vi "Martins HOT interface.vi"() -> ()   [LabVIEW 2011]
uses:
  Sub VIs/Trap cluster.ctl
  <vilib>/Utility/inputDevices.llb/closeKeyboard.vi
  <vilib>/Utility/inputDevices.llb/keyboardAcquire.vi
  <vilib>/Utility/file.llb/Write To Spreadsheet File (DBL).vi
  <vilib>/vision/driver/NI_Vision_Acquisition_Software.lvlib
panel:
  in  "e_desired":sgl=0.5
  in  "Apply Corrections":bool
  in  "View Licence":bool
  in  "ok":bool caption="Mark the center of \nthe spot using the \nzoom and the point\ntool, then click this \nbutton"
  in  "Stop program":bool
  in  "Updating trap cluster":bool=TRUE
  out "Camera enabled":bool
  out "SLM enabled":bool
  in  "Run calibration":bool
  in  "Hologram generation":cluster{"Method":i32, "Iterations":i32}={"Method"=0, "Iterations"=10} {"Method" items=["Lenses & Gratings (3D)", " Gerchberg-Saxton (3D)", "Gerchberg-Saxton FFT (2D)"]}
  in  "Show image":bool=TRUE
  in  "Follow traps":bool=TRUE
  in  "Purge data":bool
  in  "ROI size":dbl=2.0 min=2.0 step=2.0
  in  "Save data":bool
  in  "Video tracking":bool
  in  "Display hologram\nand computed \nimage plane":bool
  in  "ROI":T1={"Global Rectangle"=[309, 286, 371, 364], "Contours"=[{"Contour Type"=0, "ROI Type"=1, "Points"=[370, 286]}, {"Contour Type"=0, "ROI Type"=1, "Points"=[351, 363]}, {"Contour Type"=0, "ROI Type"=1, "Points"=[309, 315]}]}
  out "Image":T2(plugin-control)
  out "Calculated image plane":dbl[][](graph)
  in  "G":bool[](array[boolean])=[FALSE, FALSE, FALSE]
  out "Current trap pos":T3={"X (IMAQ)"=[57.0, 561.4247207088292, 45.0], "Y (IMAQ)"=[160.0, 450.3470670604607, 127.0], "Z"=[0.0, 0.0, 0.0], "Amplitudes"=[10.0, 10.0, 10.0], "Trap number"=[0, 1, 2], "ROI number"=[0, 1, 2], "Number of traps"=3, "Group"=[]}
  out "NI Vision error":errorcluster
  out "CUDA/SLM error":errorcluster
  in  "Cancel calibration":bool
  in  "Skip step if \ntimed out":bool
  in  "Display path":bool=TRUE
  out "Average step time (ms)":dbl
  in  "Step time \n(ms)":u32=10
  in  "Pause":bool
  in  "cancel path":bool
  out "Step skipped":bool
  in  "Path controls":T4={"follow path"=FALSE, "Step length"=1.0, "Arrive \nsimultaneously"=TRUE, "Synchronize traps"=FALSE, "Add current \npositions to path"=FALSE}
  in  "Create path":bool
  out "#":i32[](array[numeric])=[0, 1, 2]
  in  "Group \nTraps":bool
  in  "Move \nHandle":bool
  out "Displayed Hologram":u8[][](graph)
  in  "Coordinate mapping \n(IMAQ to SLM)":T5={"sX"=-256.0, "sY"=-256.0, "sZ"=0.0, "cX"=0.5, "cY"=0.5, "cZ"=1.0}
  in  "Switch X/Y":bool
  in  "I":dbl[](array[numeric])=[10.0, 10.0, 10.0]
  in  "Z":dbl[](array[numeric])=[0.0, 0.0, 0.0]
  # "Martin\nPersson 2011"
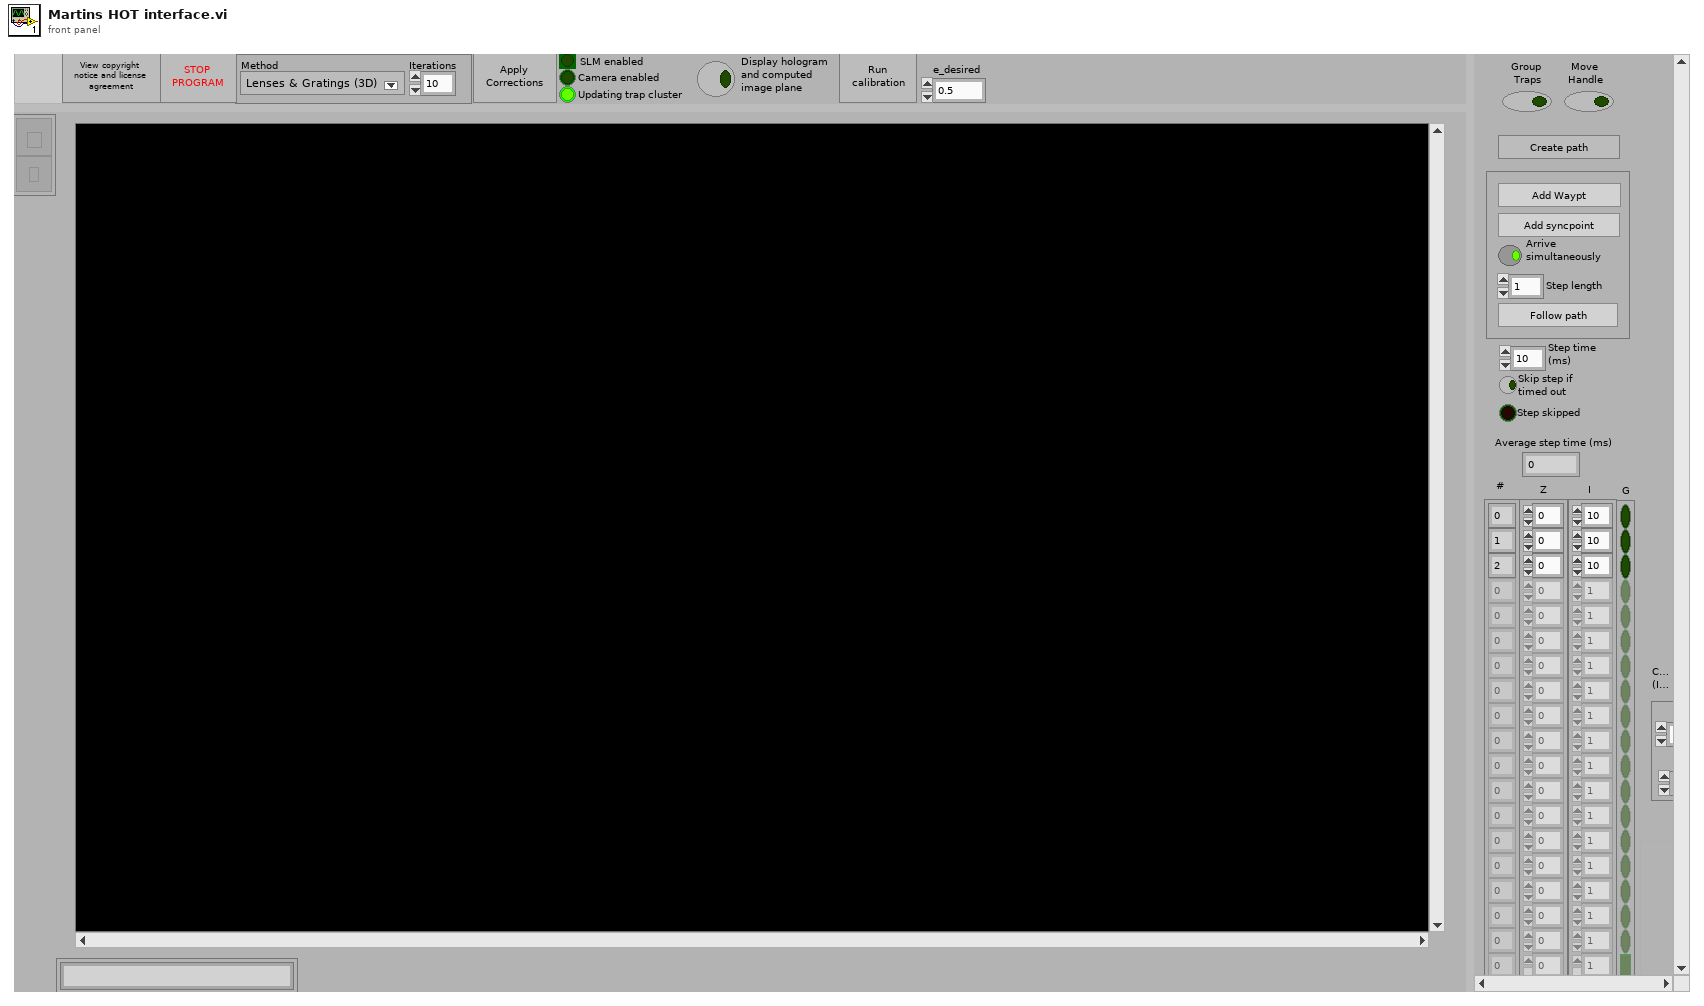
[diagram p1: front panel]
types:
  T1 = cluster{"Global Rectangle":i32[], "Contours":cluster{"Contour Type":u32, "ROI Type":u32, "Points":i32[]}[]}
  T2 = typedef "IMAQ Image.ctl" = refnum<image>
  T3 = typedef "Trap cluster.ctl" = cluster{"X (IMAQ)":dbl[], "Y (IMAQ)":dbl[], "Z":dbl[], "Amplitudes":dbl[], "Trap number":i32[], "ROI number":i32[], "Number of traps":i32, "Group":bool[]}
  T4 = cluster{"follow path":bool, "Step length":dbl, "Arrive \nsimultaneously":bool, "Synchronize traps":bool, "Add current \npositions to path":bool}
  T5 = cluster{"sX":dbl, "sY":dbl, "sZ":dbl, "cX":dbl, "cY":dbl, "cZ":dbl}
  T6 = cluster{"Centroid X":dbl[], "Centroid Y":dbl[], "Acquired Buffer Number":u32}
  T7 = typedef "IMAQdx.ctl" = refnum<k21>
  T8 = typedef "Image Type" = u32
  T9 = enum16{"0", "1", "2", "3", "4", "5", "6", "7", "8", "9", "A", "B", "C", "D", "E", "F", "G", "H", "I", "J", "K", "L", "M", "N", "O", "P", "Q", "R", "S", "T", "U", "V", "W", "X", "Y", "Z", "F1", "F2", "F3", "F4", "F5", "F6", "F7", "F8", "F9", "F10", "F11", "F12", "F13", "F14", "F15", "ADD", "BACK", "BACKSLASH", "CAPITAL", "COMMA", "DECIMAL", "DELETE", "DIVIDE", "DOWN", "END", "EQUALS", "ESCAPE", "GRAVE (`)", "HOME", "INSERT", "LBRACKET", "LCONTROL", "LEFT", "L ALT", "LSHIFT", "LWIN", "MINUS", "MULTIPLY", "NEXT", "NUMLOCK", "NUMPAD_0", "NUMPAD_1", "NUMPAD_2", "NUMPAD_3", "NUMPAD_4", "NUMPAD_5", "NUMPAD_6", "NUMPAD_7", "NUMPAD_8", "NUMPAD_9", "PAUSE", "PERIOD", "PRIOR (PG UP)", "RBRACKET", "RCONTROL", "RETURN", "RIGHT", "R ALT", "RSHIFT", "RWIN", "SCROLL", "SEMICOLON", "SLASH", "SPACE", "SUBTRACT", "TAB", "UP", "ENTER (num pad)", "' (quote)"}[]
  T10 = typedef "LVRectTypeDef.ctl" = cluster{"left":i16, "top":i16, "right":i16, "bottom":i16}
  T11 = cluster{dbl[], dbl[], "Acquired Buffer Number":u32}
  T12 = cluster{"Centroid X":dbl[], "Centroid Y":dbl[], "Acquired Buffer Number":u32}[]
  T13 = cluster{"Contour Type":u32, "ROI Type":u32, "Points":i32[]}[]
  T14 = cluster{"Contour Type":u32, "ROI Type":u32, "Points":i32[]}
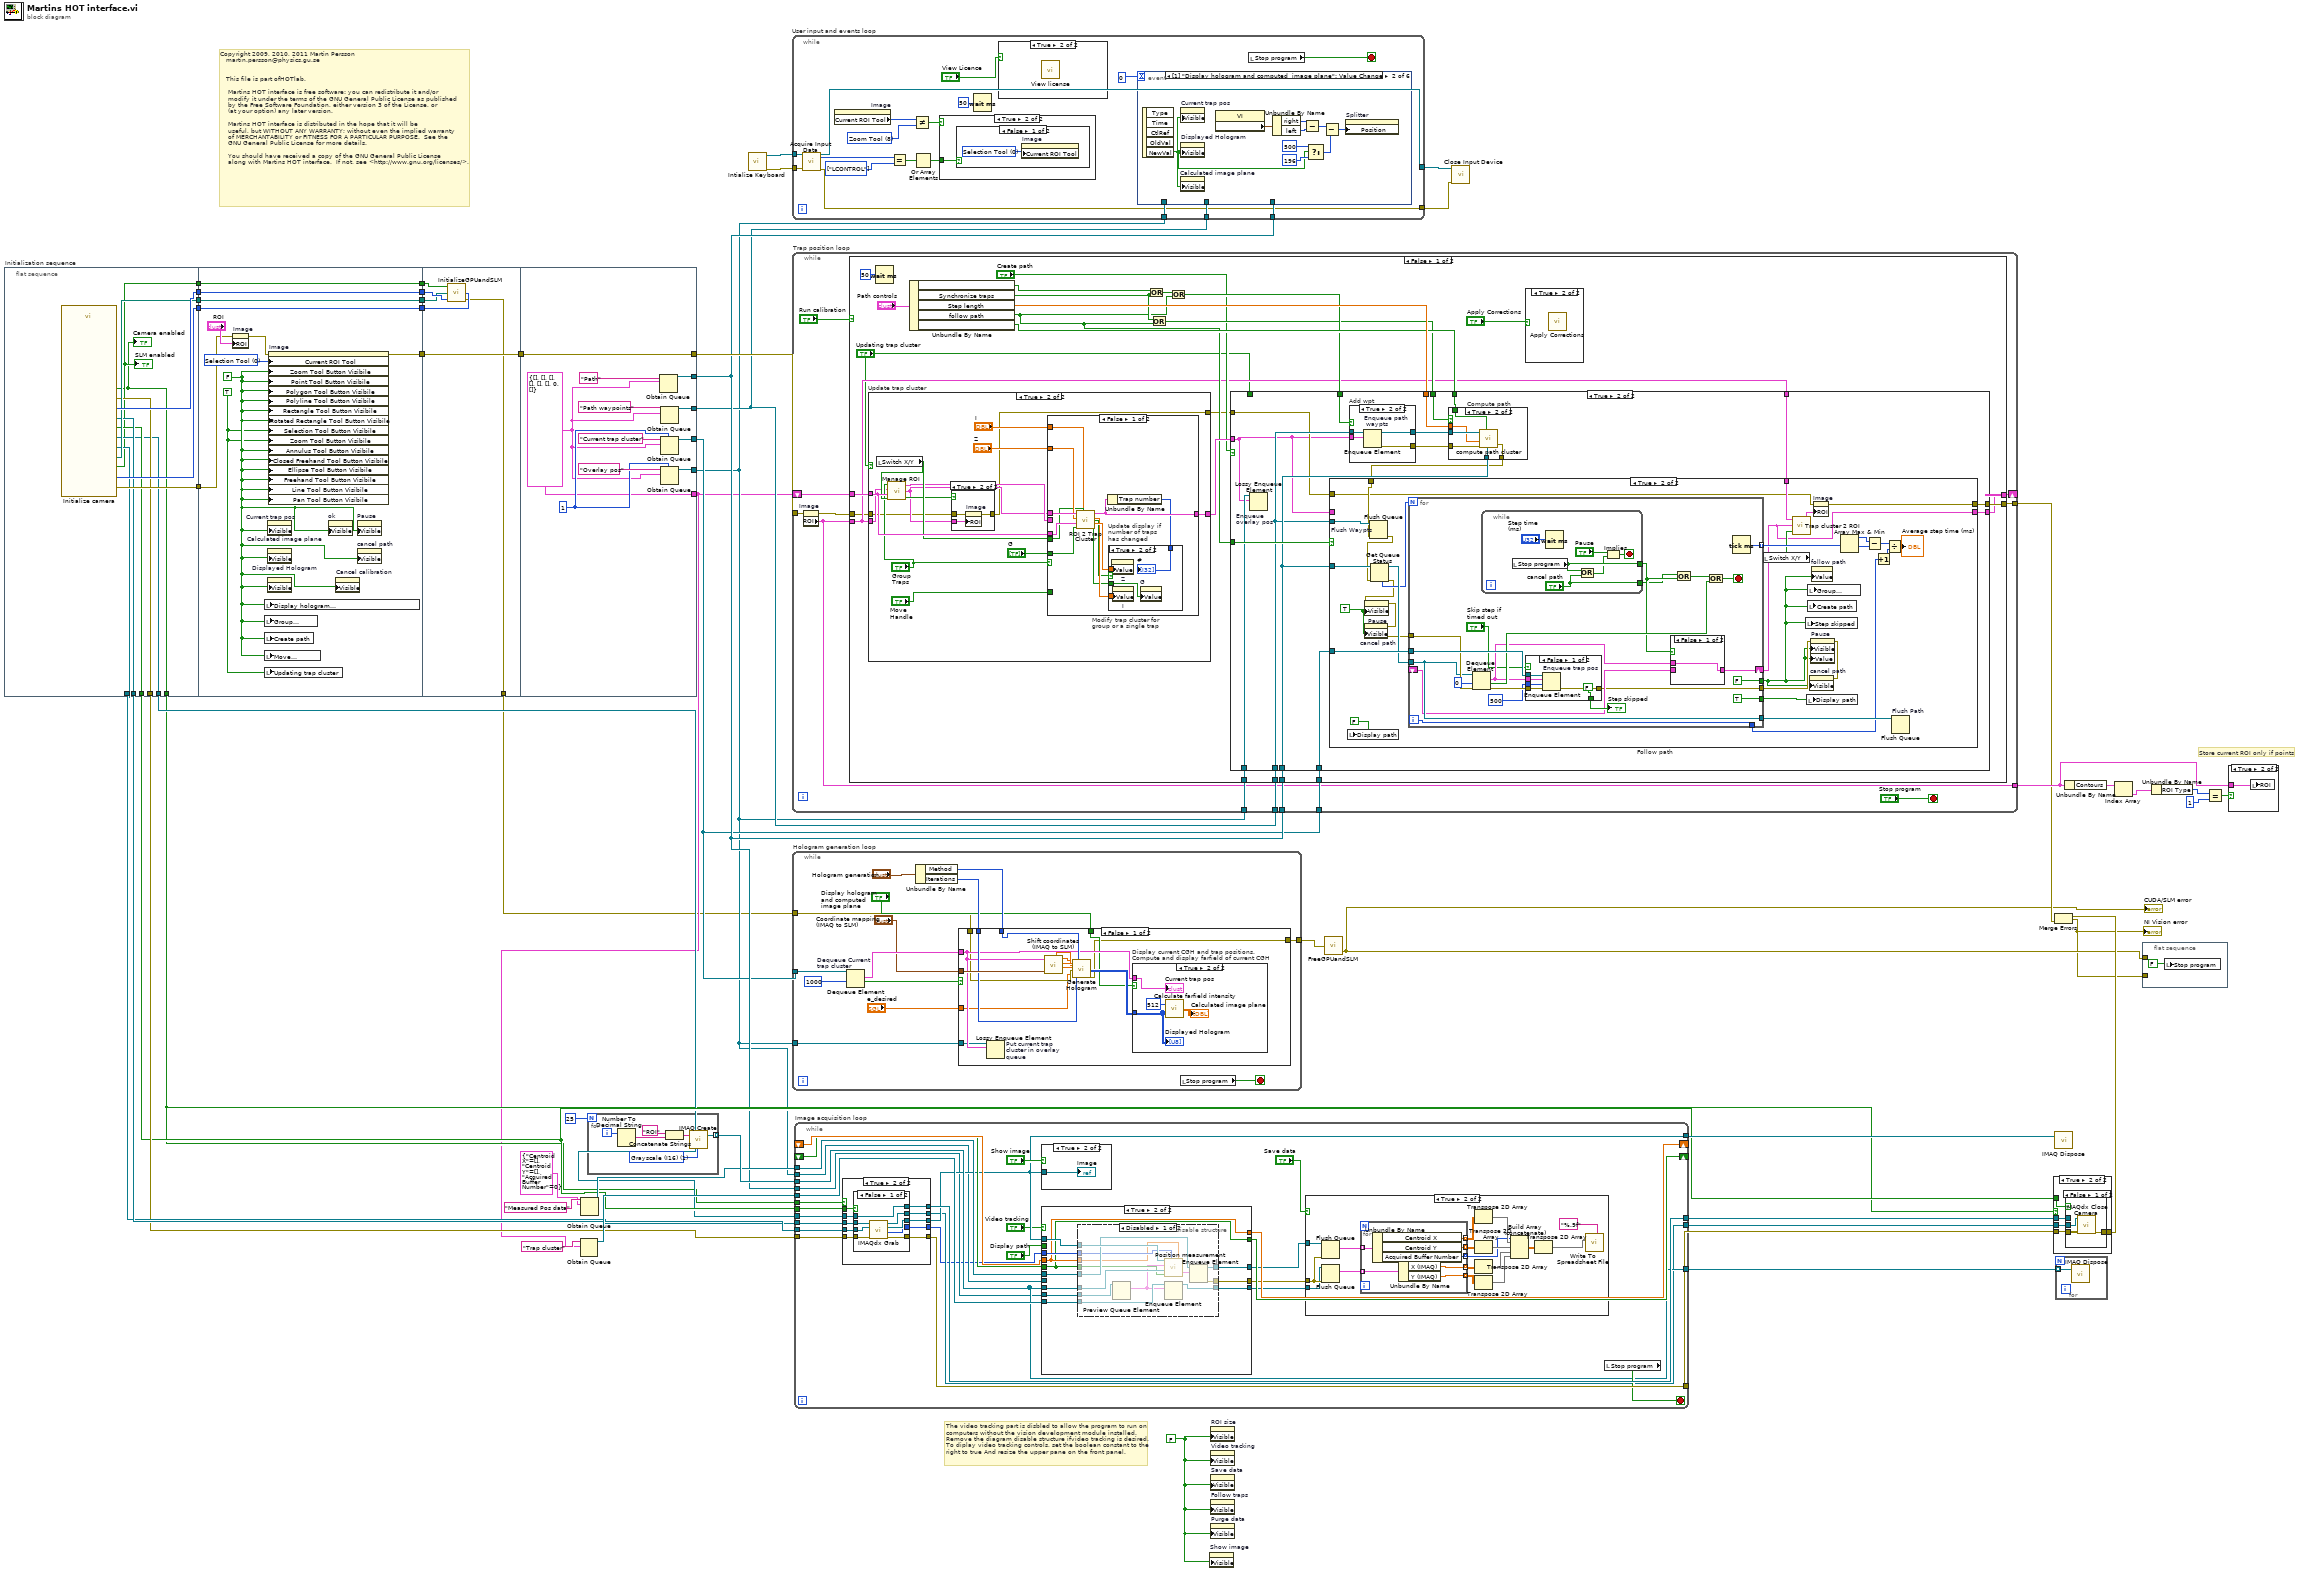
[diagram p0: block diagram]
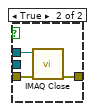
[diagram p3: hidden frame]
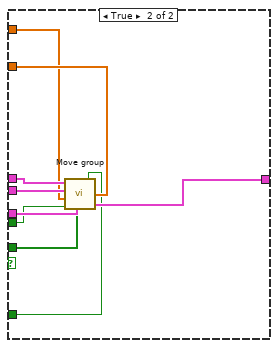
[diagram p10: hidden frame]
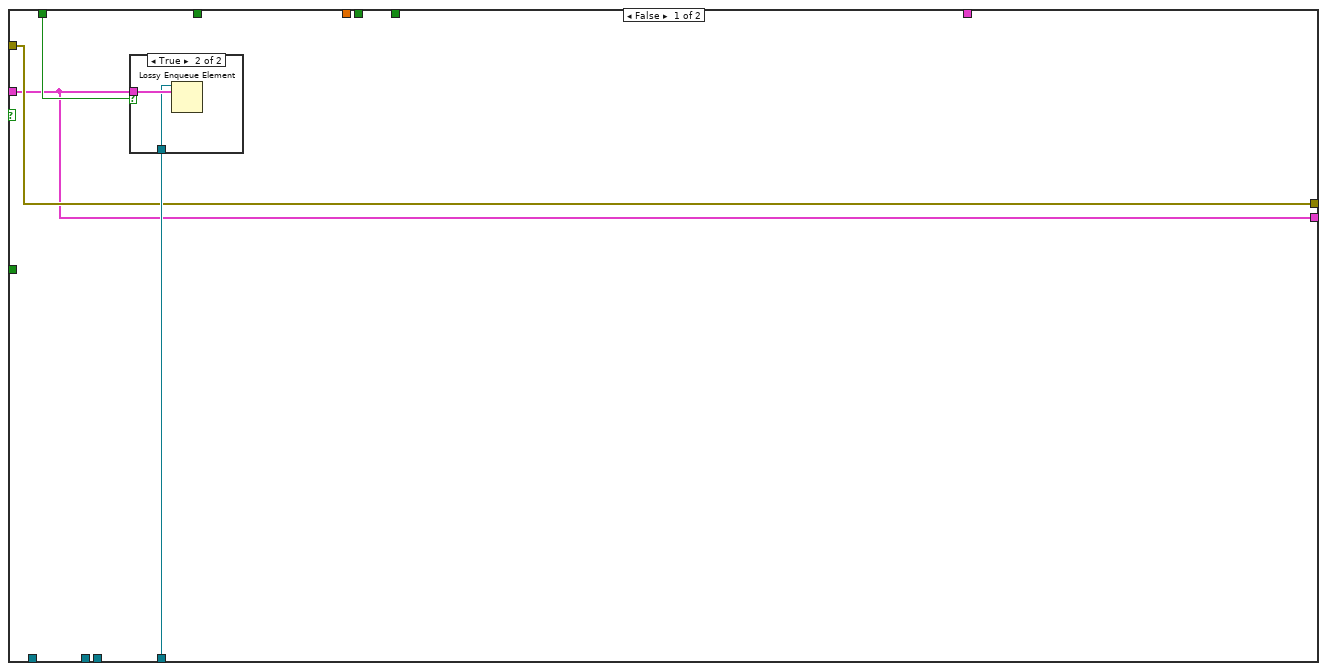
[diagram p11: hidden frame]
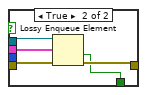
[diagram p14: hidden frame]
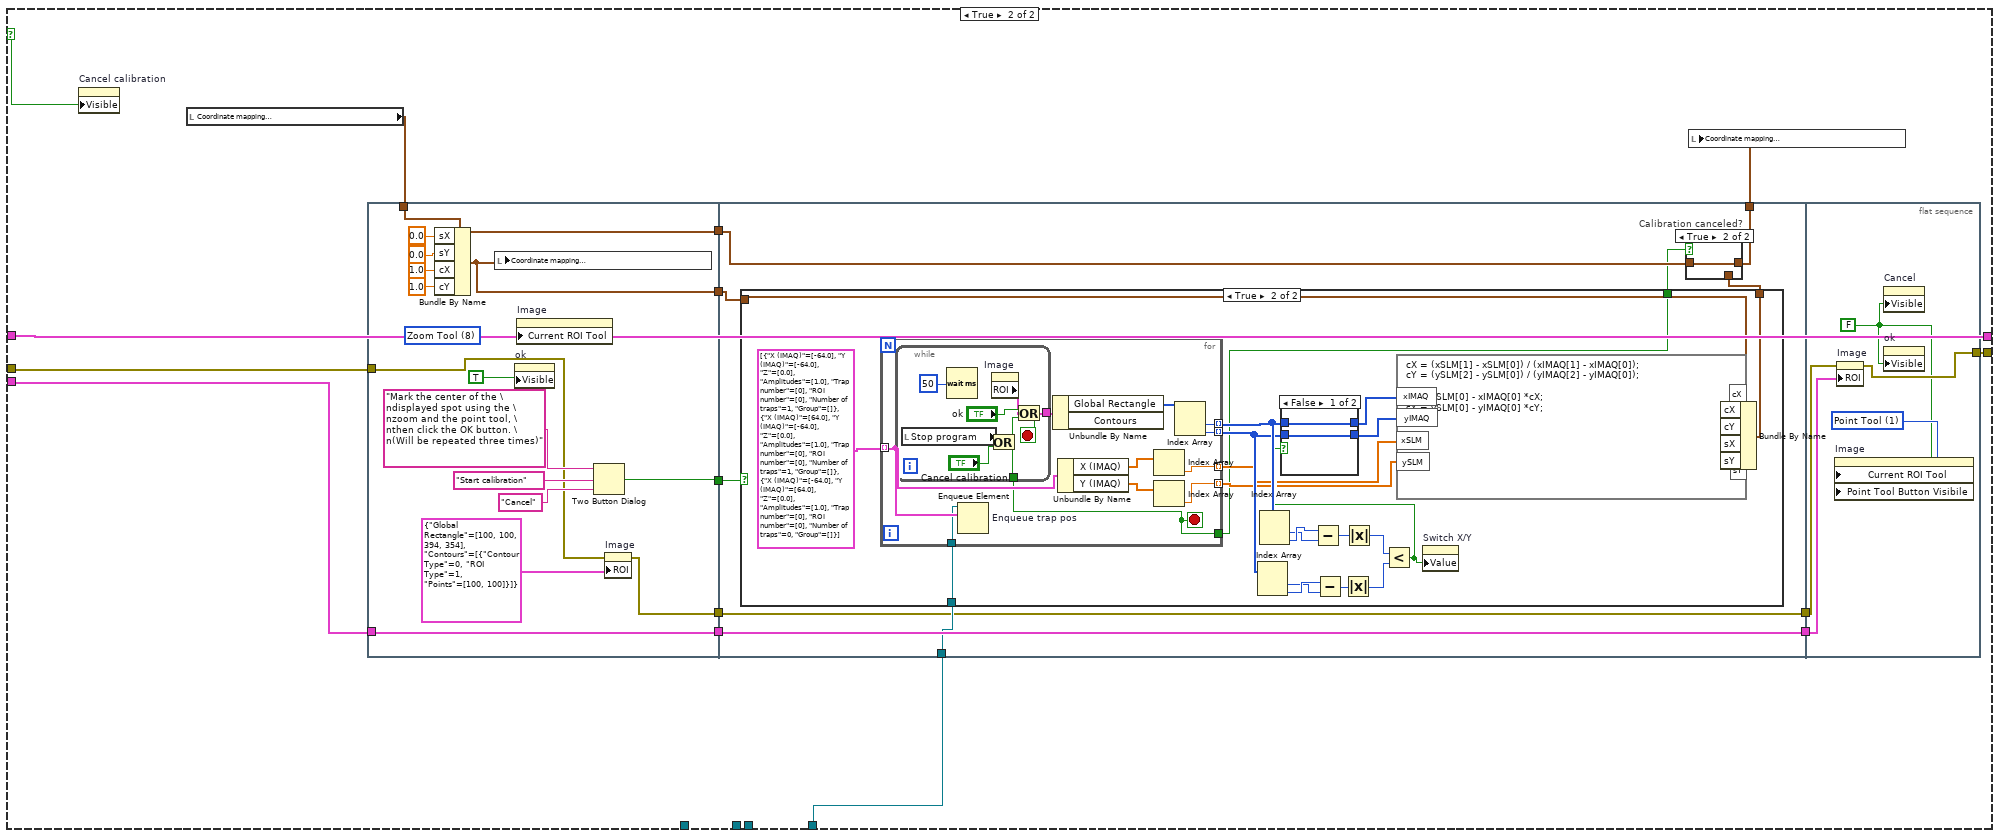
[diagram p18: hidden frame]
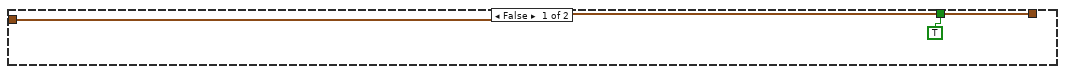
[diagram p20: hidden frame]
diagram:
  w39 = FALSE ("Visible")
  # "Copyright 2009, 2010, 2011 Martin Persson \n   martin.persson@physics.gu.se\n\n\n   This file is part ofHOTlab.\n\n    Martins HOT interface is free software: you can redistribute it and/or \n    modify it under the terms of the GNU General Public License as published \n    by the Free Software Foundation, either version 3 of the License, or\n    (at your option) any later version.\n\n    Martins HOT interface is distributed in the hope that it will be \n    useful, but WITHOUT ANY WARRANTY; without even the implied warranty\n    of MERCHANTABILITY or FITNESS FOR A PARTICULAR PURPOSE.  See the\n    GNU General Public License for more details.\n\n    You should have received a copy of the GNU General Public License\n    along with Martins HOT interface.  If not, see <http://www.gnu.org/licenses/>."
  # "Store current ROI only if points"
  # "The video tracking part is disbled to allow the program to run on\ncomputers without the vision development module installed. \nRemove the diagram disable structure ifvideo tracking is desired. \nTo diplay video tracking controls, set the boolean constant to the \nright to true And resize the upper pane on the front panel."
  n1 = flat-sequence "Initialization sequence" {
    tunnel: [w54] -> w24
    tunnel: [w63] -> w23
    tunnel: [w62] -> w22
    tunnel: [w61] -> w21
    tunnel: [w60] -> w20
    tunnel: [w59] -> w18
    tunnel: [w58] -> w17
    tunnel: [w57] -> w16
    tunnel: [w56] -> w15
    tunnel: [w55] -> w14
    tunnel: [w53] -> w13
    tunnel: w24 -> [w71]
    tunnel: w23 -> [w69]
    tunnel: w22 -> [w74]
    tunnel: w21 -> [w73]
    tunnel: w20 -> [w72]
    tunnel: [w71] -> w7
    tunnel: [w64] -> w6
    tunnel: [w74] -> w4
    tunnel: [w73] -> w3
    tunnel: [w72] -> w2
    tunnel: w7 -> [w77]
    tunnel: w6 -> [w80]
    tunnel: [w80] -> w5
    tunnel: w4 -> [w78]
    tunnel: w3 -> [w79]
    tunnel: w2 -> [w76]
    tunnel: [w75] -> w1
    tunnel: [w91] -> w19
    tunnel: w5 -> [w91]
    tunnel: [w89] -> w12
    tunnel: [w87] -> w11
    tunnel: [w85] -> w10
    tunnel: [w84] -> w9
    tunnel: [w81] -> w8
    frame #0 {
      n2 = call "Initialize camera.vi"() -> ("CUDA device ID"=w61:i32, "IMAQdx Session Out"=w58:T7, "TrueFrame out"=w62:i32, "IMAQ camera"=w56:bool, "Image reference out"=w59:T2, "SLM enabled"=w54:bool, "Camera enabled"=w53:bool, "Vision error out"=w63:errorcluster, "LUT path out"=w60:path, "IMAQ Session Out"=w55:refnum<k11>, "Camera error"=w57:errorcluster)  [unwired: 5 in]
      "Camera enabled" <- w53
      "SLM enabled" <- w54
    }
    frame #1 {
      w67 = TRUE ("ROI Tool Buttons Visibile:Zoom Tool Button Visible")
      w68 = FALSE ("ROI Tool Buttons Visibile:Zoom Tool Button Visible")
      w66 = u32 0 items=["Zoom Tool"=8, "Selection Tool"=0, "Pan Tool"=9, "Point Tool"=1, "Line Tool"=2, "Rectangle Tool"=3, "Rotated Rectangle Tool"=12, "Polyline Tool"=10, "Polygon Tool"=5, "Freehand Tool"=11, "Closed Freehand Tool"=6, "Ellipse Tool"=4, "Annulus Tool"=7] ("Current ROI Tool")
      n3 = property on="Image" class="ImageControl"(error in=w69, "ROI"="ROI") -> (error out=w65:errorcluster)  [unwired: 1 in, 1 out]
      n4 = local write "Display hologram\nand computed \nimage plane"(w68) -> ()
      n5 = local write "Group \nTraps"(w68) -> ()
      n6 = local write "Create path"(w68) -> ()
      n7 = local write "Move \nHandle"(w68) -> ()
      n8 = local write "Updating trap cluster"(w67) -> ()
      n9 = property on="Current trap pos" class="Clust (strict)"("Visible"=w68) -> ()  [unwired: 2 in, 2 out]
      n10 = property on="Calculated image plane" class="IntGraph (strict)"("Visible"=w68) -> ()  [unwired: 2 in, 2 out]
      n11 = property on="Displayed Hologram" class="IntGraph (strict)"("Visible"=w68) -> ()  [unwired: 2 in, 2 out]
      n12 = property on="Image" class="ImageControl"(error in=w65, "Current ROI Tool"=w66, "Zoom Tool Button Visibile"=w68, "Point Tool Button Visibile"=w68, "Polygon Tool Button Visibile"=w68, "Polyline Tool Button Visibile"=w68, "Rectangle Tool Button Visibile"=w68, "Rotated Rectangle Tool Button Visibile"=w68, "Selection Tool Button Visibile"=w67, "Zoom Tool Button Visibile"=w67, "Annulus Tool Button Visibile"=w68, "Closed Freehand Tool Button Visibile"=w68, "Ellipse Tool Button Visibile"=w68, "Freehand Tool Button Visibile"=w68, "Line Tool Button Visibile"=w68, "Pan Tool Button Visibile"=w68) -> (error out=w64:errorcluster)  [unwired: 1 in, 1 out]
      n13 = property on="ok" class="Bool"("Visible"=w68) -> ()  [unwired: 2 in, 2 out]
      n14 = property on="Cancel calibration" class="Bool"("Visible"=w68) -> ()  [unwired: 2 in, 2 out]
      n15 = property on="Pause" class="Bool (strict)"("Visible"=w68) -> ()  [unwired: 2 in, 2 out]
      n16 = property on="cancel path" class="Bool"("Visible"=w68) -> ()  [unwired: 2 in, 2 out]
    }
    frame #2 {
      n17 = call "InitializeGPUandSLM.vi"("TrueFrame"=w78, "deviceId"=w79, "Path to LUT file"=w76, "SLM enabled"=w77) -> ("CUDA/SLM error"=w75:errorcluster)  [unwired: 1 out]
    }
    frame #3 {
      w82 = 1 ("max queue size (-1, unlimited)")
      w81 = T3 {"X (IMAQ)"=[], "Y (IMAQ)"=[], "Z"=[], "Amplitudes"=[], "Trap number"=[], "ROI number"=[], "Number of traps"=0, "Group"=[]} ("output cluster 2")
      n18 = Obtain Queue(name (unnamed)="Path", element data type=w81) -> (queue out=w89:refnum<queue>)  [unwired: 3 in, 2 out]
      n19 = Obtain Queue(name (unnamed)="Path waypoints", element data type=w81) -> (queue out=w87:refnum<queue>)  [unwired: 3 in, 2 out]
      n20 = Obtain Queue(max queue size (-1, unlimited)=w82, name (unnamed)="Current trap cluster", element data type=w81) -> (queue out=w85:refnum<queue>)  [unwired: 2 in, 2 out]
      n21 = Obtain Queue(max queue size (-1, unlimited)=w82, name (unnamed)="Overlay pos", element data type=w81) -> (queue out=w84:refnum<queue>)  [unwired: 2 in, 2 out]
    }
  }
  n22 = Obtain Queue(name (unnamed)="Trap cluster", element data type=w8) -> (queue out=w44:refnum<queue>)  [unwired: 3 in, 2 out]
  n23 = Obtain Queue(name (unnamed)="Measured Pos data", element data type=T6 {"Centroid X"=[], "Centroid Y"=[], "Acquired Buffer Number"=0} ("output cluster 2")) -> (queue out=w47:refnum<queue>)  [unwired: 3 in, 2 out]
  n24 = for {
    N: 25 -> [_]
    tunnel: [w97] -> w49 mode=indexing
    i -> [w93]
    w95 = T8 1 items=["Grayscale (U8)", "Grayscale (I16)", "Grayscale (SGL)", "Complex (CSG)", "RGB (U32)", "HSL (U32)", "RGB (U64)", "Grayscale (U16)"] ("Image Type")
    n25 = Number To Decimal String(number=w93) -> (decimal integer string=w92:string)  [unwired: 1 in]
    n26 = Concatenate Strings("ROI" ("Image Name"), w92) -> (w94:string)
    n27 = call "IMAQ Create"("Image Name"=w94, "Image Type"=w95) -> ("New Image"=w97:T2)  [unwired: 3 in, 1 out]
  }
  n28 = call <vilib>:"Intialize Keyboard.vi"() -> ("error out"=w26:errorcluster, "device ID"=w52:refnum<k1>)  [unwired: 1 in, 9 out]
  n29 = while "User input and events loop" {
    tunnel: w52 -> [w115]
    tunnel: w9 -> [w104]
    tunnel: w11 -> [w103]
    tunnel: w12 -> [w102]
    tunnel: [w101] -> w27
    tunnel: w26 -> [w100]
    tunnel: [w99] -> w25
    stop <- w107 stop-if-true
    w112 = u32 8 items=["Zoom Tool"=8, "Selection Tool"=0, "Pan Tool"=9, "Point Tool"=1, "Line Tool"=2, "Rectangle Tool"=3, "Rotated Rectangle Tool"=12, "Polyline Tool"=10, "Polygon Tool"=5, "Freehand Tool"=11, "Closed Freehand Tool"=6, "Ellipse Tool"=4, "Annulus Tool"=7] ("Current ROI Tool")
    w109 = T9 [enum."LCONTROL"] items=["0", "1", "2", "3", "4", "5", "6", "7", "8", "9", "A", "B", "C", "D", "E", "F", "G", "H", "I", "J", "K", "L", "M", "N", "O", "P", "Q", "R", "S", "T", "U", "V", "W", "X", "Y", "Z", "F1", "F2", "F3", "F4", "F5", "F6", "F7", "F8", "F9", "F10", "F11", "F12", "F13", "F14", "F15", "ADD", "BACK", "BACKSLASH", "CAPITAL", "COMMA", "DECIMAL", "DELETE", "DIVIDE", "DOWN", "END", "EQUALS", "ESCAPE", "GRAVE (`)", "HOME", "INSERT", "LBRACKET", "LCONTROL", "LEFT", "L ALT", "LSHIFT", "LWIN", "MINUS", "MULTIPLY", "NEXT", "NUMLOCK", "NUMPAD_0", "NUMPAD_1", "NUMPAD_2", "NUMPAD_3", "NUMPAD_4", "NUMPAD_5", "NUMPAD_6", "NUMPAD_7", "NUMPAD_8", "NUMPAD_9", "PAUSE", "PERIOD", "PRIOR (PG UP)", "RBRACKET", "RCONTROL", "RETURN", "RIGHT", "R ALT", "RSHIFT", "RWIN", "SCROLL", "SEMICOLON", "SLASH", "SPACE", "SUBTRACT", "TAB", "UP", "ENTER (num pad)", "' (quote)"] ("keys pressed")
    n30 = call-poly <vilib>:"Acquire Input Data.vi"("device ID"=w115, "error in (no error)"=w100) -> ("device ID"=w101:refnum<k1>, "keys pressed"=w108:T9, "error out"=w99:errorcluster)  [unwired: 15 out]
    n31 = property on="Image" class="ImageControl"() -> ("Current ROI Tool"=w111:u32)  [unwired: 2 in, 2 out]
    n32 = Equal?(x=w108, y=w109) -> (x = y?=w110:bool[])
    n33 = Not Equal?(x=w111, y=w112) -> (x != y?=w113:bool)
    n34 = Or Array Elements(Boolean array=w110) -> (logical OR=w114:bool)
    n35 = case shown="True" w113 {
      tunnel: w114 -> [_ w136]
      frame False {
      }
      frame True {
        n36 = case shown="False" w136 {
          frame False {
            w137 = u32 0 items=["Zoom Tool"=8, "Selection Tool"=0, "Pan Tool"=9, "Point Tool"=1, "Line Tool"=2, "Rectangle Tool"=3, "Rotated Rectangle Tool"=12, "Polyline Tool"=10, "Polygon Tool"=5, "Freehand Tool"=11, "Closed Freehand Tool"=6, "Ellipse Tool"=4, "Annulus Tool"=7] ("Current ROI Tool")
            n37 = property on="Image" class="ImageControl"("Current ROI Tool"=w137) -> ()  [unwired: 2 in, 2 out]
          }
          frame True {
            w138 = u32 1 items=["Zoom Tool"=8, "Selection Tool"=0, "Pan Tool"=9, "Point Tool"=1, "Line Tool"=2, "Rectangle Tool"=3, "Rotated Rectangle Tool"=12, "Polyline Tool"=10, "Polygon Tool"=5, "Freehand Tool"=11, "Closed Freehand Tool"=6, "Ellipse Tool"=4, "Annulus Tool"=7] ("Current ROI Tool")
            n38 = property on="Image" class="ImageControl"("Current ROI Tool"=w138) -> ()  [unwired: 2 in, 2 out]
          }
        }
      }
    }
    n39 = Wait (ms)(milliseconds to wait=u32 50) -> ()  [unwired: 1 out]
    n40 = case shown="True" "View Licence" {
      frame False {
      }
      frame True {
        n41 = call "View license.vi"() -> ()  [unwired: 1 in]
      }
    }
    n42 = event shown="[1] \"Display hologram\nand computed \nimage plane\": Value Change" {
      selector: _ -> [_ _ _ _ _ _]
      dyn-events: _ -> [_ _ _ _ _ _]
      timeout: 0 -> [_ _ _ _ _ _]
      tunnel: w104 -> [_ _ w126 _ _ _]
      tunnel: w103 -> [_ _ w125 _ _ _]
      tunnel: w102 -> [_ _ w129 _ _ _]
      event Timeout {
        n43 = event-data() -> ()  [unwired: 1 in, 2 out]
      }
      event "Display hologram\nand computed \nimage plane": Value Change {
        n44 = event-data() -> ("NewVal"=w117:bool)  [unwired: 1 in, 4 out]
        n45 = property on="Current trap pos" class="Clust (strict)"("Visible"=w117) -> ()  [unwired: 2 in, 2 out]
        n46 = property on="Displayed Hologram" class="IntGraph (strict)"("Visible"=w117) -> ()  [unwired: 2 in, 2 out]
        n47 = property on="Calculated image plane" class="IntGraph (strict)"("Visible"=w117) -> ()  [unwired: 2 in, 2 out]
        n48 = property on="Property Node" class="VI"() -> ("Front Panel.WinBounds"=w124:T10)  [unwired: 2 in, 2 out]
        n49 = Unbundle By Name(w124) -> ("right"=w123:i16, "left"=w122:i16)
        n50 = Subtract(x=w123, y=w122) -> (x-y=w121:i16)
        n51 = Select(t=i16 500 ("x-y"), s=w117, f=i16 196 ("x-y")) -> (s? t:f=w116:i16)
        n52 = Subtract(x=w121, y=w116) -> (x-y=w120:i16)
        n53 = property on="Splitter" class="Splitter"("Position"=w120) -> ()  [unwired: 2 in, 2 out]
      }
      event "Create path": Value Change {
        n54 = event-data() -> ()  [unwired: 1 in, 5 out]
        n55 = property on="follow path" class="Bool (strict)"("Value"=FALSE) -> ()  [unwired: 2 in, 2 out]
        n56 = Flush Queue "Flush path \nwaypt queue"(queue=w125) -> ()  [unwired: 1 in, 3 out]
        n57 = Preview Queue Element(queue=w126) -> (element=w127:T3, error out=w130:errorcluster)  [unwired: 2 in, 2 out]
        n58 = Flush Queue "Flush path queue"(queue=w129) -> (queue out=w128:refnum<queue>)  [unwired: 1 in, 2 out]
        n59 = Enqueue Element "Enqueue current \ntrap pos in path"(queue=w128, element=w127) -> ()  [unwired: 2 in, 3 out]
        n60 = Enqueue Element "Enqueue current \ntrap pos in path \nwaypts"(queue=w125, element=w127, error in (no error)=w130) -> ()  [unwired: 1 in, 3 out]
      }
      event "cancel path": Value Change {
        n61 = event-data() -> ()  [unwired: 1 in, 5 out]
        n62 = local write "Create path"(FALSE ("Visible")) -> ()
      }
      event "Image", "Group \nTraps", "Z", "I", "Coordinate mapping \n(IMAQ to SLM)": Mouse Down {
        n63 = event-data() -> ()  [unwired: 1 in, 7 out]
        n64 = local write "Updating trap cluster"(TRUE ("Update trap positions")) -> ()
      }
      event "Group \nTraps", "Z", "I", "Image", "Coordinate mapping \n(IMAQ to SLM)": Mouse Up {
        n65 = event-data() -> ()  [unwired: 1 in, 7 out]
        n66 = flat-sequence {
          frame #0 {
            n67 = Wait (ms)(milliseconds to wait=u32 100) -> ()  [unwired: 1 out]
          }
          frame #1 {
            n68 = local write "Updating trap cluster"(FALSE ("Update trap positions")) -> ()
          }
        }
      }
    }
    n69 = local read "Stop program"() -> (w107:bool)
  }
  n70 = while "Trap position loop" {
    tunnel: w11 -> [w150]
    tunnel: w12 -> [w147]
    shift-right: [w149] -> _
    shift-left: w8 -> [w142]
    tunnel: w10 -> [w148]
    tunnel: w9 -> [w145]
    tunnel: [w144] -> w33
    tunnel: w19 -> [w141]
    tunnel: [w139] -> w31
    stop <- "Stop program" stop-if-true
    n71 = property on="Image" class="ImageControl"(error in=w141) -> (error out=w140:errorcluster, "ROI"=w144:T1)  [unwired: 1 in, 1 out]
    n72 = case shown="False" "Run calibration" {
      selector: "Run calibration" -> [_ w328]
      tunnel: w150 -> [w174 _]
      tunnel: w142 -> [w173 w327]
      tunnel: [w152 w327] -> w149
      tunnel: w148 -> [w163 w337]
      tunnel: w147 -> [w161 _]
      tunnel: w145 -> [w158 _]
      tunnel: w144 -> [w157 w336]
      tunnel: w140 -> [w156 w332]
      tunnel: [w154 w329] -> w139
      frame False {
        n73 = case "Update trap cluster" shown="True" "Updating trap cluster" {
          tunnel: w173 -> [w176 w190]
          tunnel: [w176 w182] -> w164
          tunnel: w157 -> [_ w180]
          tunnel: w156 -> [w175 w179]
          tunnel: [w175 w178] -> w155
          frame False {
          }
          frame True {
            n74 = local read "Switch X/Y"() -> (w189:bool)
            n75 = call "Manage ROI.vi"("Switch X/Y"=w189, "Trap cluster in"=w190, "ROI in"=w180, "Group traps"="Group \nTraps") -> ("Replace ROI"=w188:bool, "ROI out"=w181:T1, "Previous ROI out"=w187:T1)
            n76 = case shown="True" w188 {
              tunnel: w181 -> [_ w194]
              tunnel: w179 -> [w191 w193]
              tunnel: [w191 w192] -> w178
              frame False {
              }
              frame True {
                n77 = property on="Image" class="ImageControl"(error in=w193, "ROI"=w194) -> (error out=w192:errorcluster)  [unwired: 1 in, 1 out]
              }
            }
            n78 = case "Modify trap cluster for \ngroup or a single trap" shown="False" "Group \nTraps" {
              tunnel: [w199 w216] -> w182
              tunnel: w181 -> [w206 w217]
              tunnel: w190 -> [w205 w219]
              tunnel: w187 -> [_ w218]
              tunnel: "Z" -> [w204 w215]
              tunnel: "Move \nHandle" -> [_ w214]
              tunnel: w189 -> [w203 w213]
              tunnel: "I" -> [w201 w212]
              tunnel: "G" -> [w196 w211]
              frame False {
                n79 = call "ROI 2 Trap Cluster.vi"("Amplitudes"=w201, "Switch X/Y"=w203, "Group"=w196, "Trap Cluster in"=w205, "Z"=w204, "ROI"=w206) -> ("Group out"=w195:bool[], "Z out"=w202:dbl[], "Amplitudes out"=w200:dbl[], "Trap Cluster Out"=w199:T3, "Update display"=w197:bool)
                n80 = Unbundle By Name(w199) -> ("Trap number"=w198:i32[])
                n81 = case "Update display if\nnumber of traps \nhas changed" shown="True" w197 {
                  tunnel: w202 -> [_ w210]
                  tunnel: w200 -> [_ w209]
                  tunnel: w198 -> [_ w208]
                  tunnel: w195 -> [_ w207]
                  frame False {
                  }
                  frame True {
                    n82 = property on="Z" class="Arr (strict)"("Value"=w210) -> ()  [unwired: 2 in, 2 out]
                    n83 = property on="I" class="Arr (strict)"("Value"=w209) -> ()  [unwired: 2 in, 2 out]
                    n84 = property on="G" class="Arr (strict)"("Value"=w207) -> ()  [unwired: 2 in, 2 out]
                    "#" <- w208
                  }
                }
              }
              frame True {
                n85 = call "Move group.vi"("New handle position in"=w217, "Trap cluster in"=w219, "Previous handle position in"=w218, "Amplitudes"=w212, "Group"=w211, "Switch X/Y"=w213, "Move handle"=w214, "Z"=w215) -> ("Trap cluster out"=w216:T3)
              }
            }
          }
        }
        n86 = Wait (ms)(milliseconds to wait=u32 50) -> ()  [unwired: 1 out]
        n87 = Unbundle By Name("Path controls") -> ("Add current \npositions to path"=w159:bool, "Synchronize traps"=w168:bool, "Step length"=w171:dbl, "follow path"=w162:bool, "Arrive \nsimultaneously"=w170:bool)
        n88 = Or(x=w159, y=w168) -> (x .or. y?=w169:bool)
        n89 = Or(x=w168, y=w162) -> (x .or. y?=w166:bool)
        n90 = Or(x=w169, y=w162) -> (x .or. y?=w167:bool)
        n91 = case shown="True" "Create path" {
          tunnel: w174 -> [_ w232]
          tunnel: w164 -> [w220 w226]
          tunnel: w171 -> [_ w241]
          tunnel: w161 -> [_ w236]
          tunnel: w170 -> [_ w240]
          tunnel: w167 -> [_ w239]
          tunnel: w166 -> [_ w238]
          tunnel: w162 -> [_ w237]
          tunnel: w163 -> [w223 w233]
          tunnel: w158 -> [_ w231]
          tunnel: w157 -> [_ w230]
          tunnel: w155 -> [w222 w229]
          tunnel: [w222 w228] -> w154
          tunnel: "Updating trap cluster" -> [w221 _]
          tunnel: [w220 w227] -> w152
          frame False {
            n92 = case shown="True" w221 {
              tunnel: w220 -> [_ w225]
              tunnel: w223 -> [_ w224]
              frame False {
              }
              frame True {
                n93 = Lossy Enqueue Element(queue=w224, element=w225) -> ()  [unwired: 1 in, 4 out]
              }
            }
          }
          frame True {
            n94 = Lossy Enqueue Element "Enqueue\noverlay pos"(queue=w231, element=w226) -> ()  [unwired: 1 in, 4 out]
            n95 = case "Add wpt" shown="True" w239 {
              tunnel: w226 -> [_ w318]
              tunnel: w232 -> [w315 w319]
              tunnel: [w315 w316] -> w242
              tunnel: [_ w317] -> w234
              frame False {
              }
              frame True {
                n96 = Enqueue Element "Enqueue path\n waypts"(queue=w319, element=w318) -> (queue out=w316:refnum<queue>, error out=w317:errorcluster)  [unwired: 2 in, 1 out]
              }
            }
            n97 = case "Compute path" shown="True" w238 {
              tunnel: w242 -> [_ w326]
              tunnel: w236 -> [_ w325]
              tunnel: w241 -> [_ w324]
              tunnel: w240 -> [_ w323]
              tunnel: [w320 w321] -> w235
              tunnel: w234 -> [w320 w322]
              frame False {
              }
              frame True {
                n98 = call "compute path cluster.vi"("path queue"=w325, "Arrive simultaeously"=w323, "error in (no error)"=w322, "Step length\n(IMAQ pixels)"=w324, "waypoint queue"=w326) -> ("error out"=w321:errorcluster)  [unwired: 2 in]
              }
            }
            n99 = case "Follow path" shown="True" w237 {
              tunnel: w236 -> [_ w271]
              tunnel: w235 -> [_ w272]
              tunnel: w233 -> [_ w274]
              tunnel: w232 -> [_ w273]
              tunnel: w230 -> [_ w270]
              tunnel: w229 -> [w244 w251]
              tunnel: [w244 w250] -> w228
              tunnel: [w243 w245] -> w227
              tunnel: w226 -> [w243 _]
              frame False {
              }
              frame True {
                w265 = TRUE ("Visible")
                n100 = local write "Display path"(FALSE ("Display path")) -> ()
                n101 = Flush Queue "Flush Waypts"(queue=w273, error in (no error)=w272) -> (error out=w264:errorcluster)  [unwired: 2 out]
                n102 = Get Queue Status(queue=w271, error in (no error)=w264) -> (queue out=w268:refnum<queue>, error out=w263:errorcluster, # elements in queue=w267:i32)  [unwired: 1 in, 5 out]
                n103 = property on="Pause" class="Bool (strict)"(error in=w263, "Visible"=w265) -> (error out=w262:errorcluster)  [unwired: 1 in, 1 out]
                n104 = property on="cancel path" class="Bool"(error in=w262, "Visible"=w265) -> (error out=w261:errorcluster)  [unwired: 1 in, 1 out]
                n105 = for {
                  N: w267 -> [_]
                  tunnel: w261 -> [w293]
                  tunnel: w274 -> [w295]
                  tunnel: w268 -> [w291]
                  tunnel: [w291] -> w266
                  tunnel: [FALSE ("Group traps")] -> w246
                  shift-right: [w282] -> w245
                  shift-left: _ -> [w284]
                  tunnel: [w281] -> w260
                  tunnel: [w278] -> w258 mode=indexing
                  tunnel: [w279] -> w254
                  tunnel: [TRUE ("Display path")] -> w252
                  i -> [w279]
                  stop <- w288 stop-if-true
                  n106 = Dequeue Element(queue=w291, timeout in ms (-1)=0, error in (no error)=w293) -> (element=w283:T3, timed out?=w287:bool, error out=w294:errorcluster)  [unwired: 1 out]
                  n107 = while {
                    tunnel: [w312] -> w285
                    tunnel: ["cancel path"] -> w280
                    stop <- w314 stop-if-true
                    n108 = local read "Stop program"() -> (w312:bool)
                    n109 = Wait (ms)(milliseconds to wait="Step time \n(ms)") -> ()  [unwired: 1 out]
                    n110 = Or(x=w312, y="cancel path") -> (x .or. y?=w310:bool)
                    n111 = Implies(1:w310, 2:"Pause") -> (0:w314:bool)
                  }
                  n112 = case shown="False" "Skip step if \ntimed out" {
                    tunnel: w295 -> [w301 w306]
                    tunnel: w294 -> [w300 w304]
                    tunnel: [FALSE ("overflow?") w302] -> w286
                    tunnel: w283 -> [w299 w305]
                    tunnel: [w298 w303] -> w281
                    tunnel: 500 ("timeout in ms (-1)") -> [w297 _]
                    frame False {
                      n113 = Enqueue Element "Enqueue trap pos"(queue=w301, element=w299, timeout in ms (-1)=w297, error in (no error)=w300) -> (error out=w298:errorcluster)  [unwired: 2 out]
                    }
                    frame True {
                      n114 = Lossy Enqueue Element(queue=w306, element=w305, error in (no error)=w304) -> (overflow?=w302:bool, error out=w303:errorcluster)  [unwired: 2 out]
                    }
                  }
                  "Step skipped" <- w286
                  n115 = case shown="False" w285 {
                    tunnel: w284 -> [_ w308]
                    tunnel: w283 -> [w307 _]
                    tunnel: [w307 w308] -> w282
                    frame False {
                    }
                    frame True {
                    }
                  }
                  n116 = Or(x=w280, y=w285) -> (x .or. y?=w290:bool)
                  n117 = Or(x=w290, y=w287) -> (x .or. y?=w288:bool)
                  n118 = Tick Count (ms)() -> (millisecond timer value=w278:u32)
                }
                n119 = local read "Switch X/Y"() -> (w248:bool)
                n120 = call "Trap cluster 2 ROI.vi"("Switch X/Y"=w248, "Trap cluster"=w245, "ROI in"=w270) -> ("ROI out"=w269:T1)
                n121 = local write "Step skipped"(w246) -> ()
                n122 = local write "Display path"(w252) -> ()
                n123 = local write "Create path"(w246) -> ()
                n124 = local write "Group \nTraps"(w246) -> ()
                n125 = property on="Pause" class="Bool (strict)"(error in=w260, "Visible"=w246, "Value"=w246) -> (error out=w259:errorcluster)  [unwired: 1 in, 1 out]
                n126 = property on="cancel path" class="Bool"(error in=w259, "Visible"=w246) -> ()  [unwired: 1 in, 2 out]
                n127 = property on="follow path" class="Bool (strict)"("Value"=w246) -> ()  [unwired: 2 in, 2 out]
                n128 = property on="Image" class="ImageControl"(error in=w251, "ROI"=w269) -> (error out=w250:errorcluster)  [unwired: 1 in, 1 out]
                n129 = Array Max & Min(array=w258) -> (max value=w257:u32, min value=w256:u32)  [unwired: 2 out]
                n130 = Subtract(x=w257, y=w256) -> (x-y=w255:u32)
                n131 = Increment(x=w254) -> (x+1=w249:i32)
                n132 = Divide(x=w255, y=w249) -> (x/y=→"Average step time (ms)":dbl)
                n133 = Flush Queue "Flush Path"(queue=w266) -> ()  [unwired: 1 in, 3 out]
              }
            }
          }
        }
        n134 = case shown="True" "Apply Corrections" {
          frame False {
          }
          frame True {
            n135 = call "Apply Corrections.vi"() -> ()  [unwired: 1 in]
          }
        }
      }
      frame True {
        n136 = property on="Cancel calibration" class="Bool"("Visible"=w328) -> ()  [unwired: 2 in, 2 out]
        n137 = local read "Coordinate mapping \n(IMAQ to SLM)"() -> (w335:T5)
        n138 = flat-sequence {
          tunnel: [w351] -> w341
          tunnel: [w353] -> w340
          tunnel: w336 -> [w351]
          tunnel: w335 -> [w345]
          tunnel: [w342] -> w334
          tunnel: [w345] -> w333
          tunnel: w332 -> [w344]
          tunnel: [w343] -> w330
          tunnel: [w366] -> w339
          tunnel: w341 -> [w366]
          tunnel: w340 -> [w360]
          tunnel: [w362] -> w338
          tunnel: w337 -> [w365]
          tunnel: w334 -> [w364]
          tunnel: w333 -> [w361]
          tunnel: [w358] -> w331
          tunnel: w330 -> [w358]
          tunnel: w339 -> [w421]
          tunnel: w331 -> [w419]
          tunnel: [w418] -> w329
          frame #0 {
            w354 = u32 8 items=["Zoom Tool"=8, "Selection Tool"=0, "Pan Tool"=9, "Point Tool"=1, "Line Tool"=2, "Rectangle Tool"=3, "Rotated Rectangle Tool"=12, "Polyline Tool"=10, "Polygon Tool"=5, "Freehand Tool"=11, "Closed Freehand Tool"=6, "Ellipse Tool"=4, "Annulus Tool"=7] ("Current ROI Tool")
            n139 = Bundle By Name(cluster=w345, "sX"=0.0, "sY"=0.0, "cX"=1.0 ("sX"), "cY"=1.0) -> (w342:T5)
            n140 = local write "Coordinate mapping \n(IMAQ to SLM)"(w342) -> ()
            n141 = property on="ok" class="Bool"("Visible"=TRUE ("ROI Tool Buttons Visibile:Zoom Tool Button Visible")) -> ()  [unwired: 2 in, 2 out]
            n142 = property on="Image" class="ImageControl"("Current ROI Tool"=w354) -> ()  [unwired: 2 in, 2 out]
            n143 = Two Button Dialog(message="Mark the center of the \ndisplayed spot using the \nzoom and the point tool, \nthen click the OK button. \n(Will be repeated three times)", 1:"Cancel" ("F button name (\"Cancel\")"), 2:"Start calibration" ("T button name (\"OK\")")) -> (T button?=w353:bool)
            n144 = property on="Image" class="ImageControl"(error in=w344, "ROI"=T1 {"Global Rectangle"=[100, 100, 394, 354], "Contours"=[{"Contour Type"=0, "ROI Type"=1, "Points"=[100, 100]}]} ("ROI 2")) -> (error out=w343:errorcluster)  [unwired: 1 in, 1 out]
          }
          frame #1 {
            n145 = case shown="True" w360 {
              tunnel: w364 -> [w370 w381]
              tunnel: [w370 w376] -> w363
              tunnel: w365 -> [_ w372]
              tunnel: [TRUE ("Stop program") w371] -> w359
              frame False {
              }
              frame True {
                n146 = for {
                  tunnel: [w408] -> w390 mode=indexing
                  tunnel: [w407] -> w389 mode=indexing
                  tunnel: T3[] [{"X (IMAQ)"=[-64.0], "Y (IMAQ)"=[-64.0], "Z"=[0.0], "Amplitudes"=[1.0], "Trap number"=[0], "ROI number"=[0], "Number of traps"=1, "Group"=[]}, {"X (IMAQ)"=[64.0], "Y (IMAQ)"=[-64.0], "Z"=[0.0], "Amplitudes"=[1.0], "Trap number"=[0], "ROI number"=[0], "Number of traps"=1, "Group"=[]}, {"X (IMAQ)"=[-64.0], "Y (IMAQ)"=[64.0], "Z"=[0.0], "Amplitudes"=[1.0], "Trap number"=[0], "ROI number"=[0], "Number of traps"=0, "Group"=[]}] -> [w405] mode=indexing
                  tunnel: [w402] -> w374 mode=indexing
                  tunnel: [w400] -> w373 mode=indexing
                  tunnel: w372 -> [w404]
                  tunnel: [w399] -> w371
                  stop <- w399 stop-if-true
                  n147 = while {
                    tunnel: [w415] -> w406
                    tunnel: [w411] -> w399
                    stop <- w413 stop-if-true
                    n148 = local read "Stop program"() -> (w412:bool)
                    n149 = Wait (ms)(milliseconds to wait=u32 50) -> ()  [unwired: 1 out]
                    n150 = Or(x=w412, y="Cancel calibration") -> (x .or. y?=w411:bool)
                    n151 = property on="Image" class="ImageControl"() -> ("ROI"=w415:T1)  [unwired: 2 in, 2 out]
                    n152 = Or(x="ok", y=w411) -> (x .or. y?=w413:bool)
                  }
                  n153 = Enqueue Element "Enqueue trap pos"(queue=w404, element=w405) -> ()  [unwired: 2 in, 3 out]
                  n154 = Unbundle By Name(w406) -> ("Global Rectangle"=w409:i32[])  [unwired: 1 out]
                  n155 = Unbundle By Name(w405) -> ("X (IMAQ)"=w403:dbl[], "Y (IMAQ)"=w401:dbl[])
                  n156 = Index Array(array=w403) -> (element=w402:dbl)  [unwired: 1 in]
                  n157 = Index Array(array=w401) -> (element=w400:dbl)  [unwired: 1 in]
                  n158 = Index Array(array=w409) -> (element #1=w408:i32, element #2=w407:i32)  [unwired: 2 in]
                }
                n159 = Index Array(array=w389) -> (element #1=w391:i32, element #2=w392:i32)  [unwired: 2 in]
                n160 = Index Array(array=w390) -> (element #1=w393:i32, element #2=w394:i32)  [unwired: 2 in]
                n161 = Subtract(x=w394, y=w393) -> (x-y=w386:i32)
                n162 = Subtract(x=w392, y=w391) -> (x-y=w384:i32)
                n163 = Absolute Value(x=w384) -> (abs(x)=w383:i32)
                n164 = Absolute Value(x=w386) -> (abs(x)=w385:i32)
                n165 = Less?(x=w385, y=w383) -> (x < y?=w382:bool)
                n166 = case shown="False" w382 {
                  tunnel: w390 -> [w396 w398]
                  tunnel: w389 -> [w395 w397]
                  tunnel: [w395 w398] -> w387
                  tunnel: [w396 w397] -> w388
                  frame False {
                  }
                  frame True {
                  }
                }
                n167 = formula code="cX = (xSLM[1] - xSLM[0]) / (xIMAQ[1] - xIMAQ[0]); \ncY = (ySLM[2] - ySLM[0]) / (yIMAQ[2] - yIMAQ[0]); \n\nsX = xSLM[0] - xIMAQ[0] *cX;\nsY = ySLM[0] - yIMAQ[0] *cY;"("xIMAQ"=w388, "yIMAQ"=w387, "xSLM"=w374, "ySLM"=w373) -> ("cX"=w380:dbl, "cY"=w379:dbl, "sX"=w378:dbl, "sY"=w377:dbl)
                n168 = property on="Switch X/Y" class="Bool (strict)"("Value"=w382) -> ()  [unwired: 2 in, 2 out]
                n169 = Bundle By Name(cluster=w381, "cX"=w380, "cY"=w379, "sX"=w378, "sY"=w377) -> (w376:T5)
              }
            }
            n170 = case "Calibration canceled?" shown="True" w359 {
              tunnel: w363 -> [w367 _]
              tunnel: [w367 w368] -> w362
              tunnel: w361 -> [_ w368]
              frame False {
              }
              frame True {
              }
            }
          }
          frame #2 {
            w417 = FALSE ("ROI Tool Buttons Visibile:Zoom Tool Button Visible")
            w420 = u32 1 items=["Zoom Tool"=8, "Selection Tool"=0, "Pan Tool"=9, "Point Tool"=1, "Line Tool"=2, "Rectangle Tool"=3, "Rotated Rectangle Tool"=12, "Polyline Tool"=10, "Polygon Tool"=5, "Freehand Tool"=11, "Closed Freehand Tool"=6, "Ellipse Tool"=4, "Annulus Tool"=7] ("Current ROI Tool")
            n171 = property on="Image" class="ImageControl"("Current ROI Tool"=w420, "Point Tool Button Visibile"=w417) -> ()  [unwired: 2 in, 2 out]
            n172 = property on="Image" class="ImageControl"(error in=w419, "ROI"=w421) -> (error out=w418:errorcluster)  [unwired: 1 in, 1 out]
            n173 = property on="Cancel" class="Bool"("Visible"=w417) -> ()  [unwired: 2 in, 2 out]
            n174 = property on="ok" class="Bool"("Visible"=w417) -> ()  [unwired: 2 in, 2 out]
          }
        }
        n175 = local write "Coordinate mapping \n(IMAQ to SLM)"(w338) -> ()
      }
    }
  }
  n176 = while "Hologram generation loop" {
    tunnel: w10 -> [w431]
    tunnel: w9 -> [w429]
    tunnel: w1 -> [w424]
    tunnel: [w423] -> w30
    stop <- w432 stop-if-true
    n177 = Dequeue Element "Dequeue Current \ntrap cluster"(queue=w431, timeout in ms (-1)=1000) -> (element=w430:T3, timed out?=w428:bool)  [unwired: 1 in, 2 out]
    n178 = Unbundle By Name("Hologram generation") -> ("Method"=w435:i32, "Iterations"=w434:i32)
    n179 = case shown="False" w428 {
      tunnel: "Coordinate mapping \n(IMAQ to SLM)" -> [w449 _]
      tunnel: "Display hologram\nand computed \nimage plane" -> [w439 _]
      tunnel: w435 -> [w443 _]
      tunnel: w434 -> [w442 _]
      tunnel: w430 -> [w441 _]
      tunnel: w429 -> [w440 _]
      tunnel: w424 -> [w438 w454]
      tunnel: [w437 w454] -> w423
      tunnel: "e_desired" -> [w436 _]
      frame False {
        n180 = Lossy Enqueue Element "Put current trap \ncluster in overlay \nqueue"(queue=w440, element=w441) -> ()  [unwired: 1 in, 4 out]
        n181 = call "Shift coordinates (IMAQ to SLM).vi"("Trap cluster"=w441, "Coordinate mapping \n(IMAQ to SLM)"=w449) -> ("X (SLM)"=w444:sgl[], "Y (SLM)"=w447:sgl[], "Intensities"=w445:sgl[], "Z (SLM)"=w446:sgl[])  [unwired: 1 in, 1 out]
        n182 = call "Generate Hologram.vi"("x"=w444, "y"=w447, "z"=w446, "spot_intensities"=w445, "CUDA/SLM error in"=w438, "e_desired"=w436, "N_iterations"=w442, "method"=w443) -> ("CGH out"=w448:u8[][], "CUDA/SLM error out"=w437:errorcluster)  [unwired: 17 in, 1 out]
        n183 = case "Display current CGH and trap positions.\nCompute and display farfield of current CGH" shown="True" w439 {
          tunnel: w448 -> [_ w452]
          tunnel: w441 -> [_ w451]
          frame False {
          }
          frame True {
            n184 = call "Calculate farfield intensity.vi"("h_pSLM"=w452, "Numeric"=512) -> ("Calculated image plane"=→"Calculated image plane":dbl[][])
            "Displayed Hologram" <- w452
            "Current trap pos" <- w451
          }
        }
      }
      frame True {
      }
    }
    n185 = local read "Stop program"() -> (w432:bool)
  }
  n186 = while "Image acquisition loop" {
    tunnel: w13 -> [w455]
    tunnel: w18 -> [w482]
    tunnel: w14 -> [w481]
    tunnel: [w480] -> w51
    tunnel: [w479] -> w50
    tunnel: w49 -> [w470]
    tunnel: w47 -> [w477]
    shift-right: [w476] -> _
    shift-left: _ -> [w475]
    tunnel: w44 -> [w474]
    shift-right: [w473] -> _
    shift-left: _ -> [w472]
    tunnel: [w470] -> w42
    tunnel: [w469] -> w41
    tunnel: [w468] -> w40
    tunnel: w17 -> [w467]
    tunnel: w15 -> [w466]
    tunnel: w9 -> [w465]
    tunnel: w12 -> [w464]
    tunnel: w16 -> [w462]
    stop <- w478 stop-if-true
    n187 = case shown="True" w455 {
      tunnel: w482 -> [w485 w496]
      tunnel: w481 -> [w484 w495]
      tunnel: [w484 w494] -> w480
      tunnel: [w483 w493] -> w479
      tunnel: [w485 w492] -> w469
      tunnel: [w486 w491] -> w468
      tunnel: w467 -> [w486 w490]
      tunnel: w466 -> [_ w489]
      tunnel: w462 -> [w483 w488]
      tunnel: [_ w487] -> w461
      frame False {
      }
      frame True {
        n188 = case shown="False" w489 {
          tunnel: w496 -> [w504 w512]
          tunnel: [w502 w511] -> w494
          tunnel: [w501 w510] -> w493
          tunnel: w495 -> [w502 w509]
          tunnel: [w503 w508] -> w492
          tunnel: [w498 w507] -> w487
          tunnel: [w500 w506] -> w491
          tunnel: w490 -> [w499 w506]
          tunnel: w488 -> [w497 w505]
          frame False {
            n189 = call <vilib>:"IMAQdx Grab.vi"("error in"=w497, "Image In"=w504, "Session In"=w499) -> ("error out"=w501:errorcluster, "Buffer Number Out"=w498:u32, "Image Out"=w503:T2, "Session Out"=w500:T7)  [unwired: 5 in]
          }
          frame True {
            n190 = call <vilib>:"IMAQ Grab Acquire.vi"("error in (no error)"=w505, "Image In"=w512, "IMAQ Session In"=w509) -> ("error out"=w510:errorcluster, "Acquired Buffer Number"=w507:u32, "Image Out"=w508:T2, "IMAQ Session Out"=w511:refnum<k11>)  [unwired: 1 in, 4 out]
          }
        }
      }
    }
    n191 = case shown="True" "Show image" {
      tunnel: w469 -> [_ w579]
      frame False {
      }
      frame True {
        "Image" <- w579
      }
    }
    n192 = case shown="True" "Video tracking" {
      tunnel: w469 -> [w522 w536]
      tunnel: w470 -> [_ w535]
      tunnel: w477 -> [w525 w534]
      tunnel: w461 -> [_ w533]
      tunnel: [w525 w532] -> w460
      tunnel: [_ w531] -> w457
      tunnel: ["ROI size" w530] -> w476
      tunnel: w475 -> [_ w530]
      tunnel: w474 -> [w524 w529]
      tunnel: [w524 w528] -> w456
      tunnel: ["Follow traps" w527] -> w473
      tunnel: w472 -> [_ w527]
      tunnel: w464 -> [w517 w526]
      tunnel: w465 -> [w516 _]
      tunnel: "Display path" -> [w514 _]
      frame False {
        n193 = Preview Queue Element(queue=w516, timeout in ms (-1)=10) -> (element=w515:T3)  [unwired: 1 in, 3 out]
        n194 = Get Queue Status(queue=w517, return elements? (F)=w514) -> (elements=w518:T3[])  [unwired: 1 in, 7 out]
        n195 = Wait (ms)(milliseconds to wait=u32 100) -> ()  [unwired: 1 out]
        n196 = call "Create trap overlay.vi"("Current trap cluster"=w515, "Image in"=w522, "ROI size"="ROI size", "Switch X/Y"="Switch X/Y", "Path"=w518) -> ()  [unwired: 1 out]
      }
      frame True {
        n197 = disable-structure shown="Disabled" {
          disable-tunnel: w536 -> [w549 _]
          disable-tunnel: w535 -> [w548 _]
          disable-tunnel: w534 -> [w547 _]
          disable-tunnel: w533 -> [w546 _]
          disable-tunnel: [w544 _] -> w532
          disable-tunnel: [w543 _] -> w531
          disable-tunnel: w530 -> [w542 _]
          disable-tunnel: w529 -> [w541 _]
          disable-tunnel: [w540 _] -> w528
          disable-tunnel: w527 -> [w539 _]
          disable-tunnel: w526 -> [w537 _]
          frame Disabled {
            n198 = Preview Queue Element(queue=w537) -> (element=w538:T3)  [unwired: 2 in, 3 out]
            n199 = call "Position measurement.vi"("Image"=w549, "Trap positions"=w538, "ROIs"=w548, "Follow traps?"=w539, "Acquired Buffer Number"=w546, "ROI size"=w542) -> ("Position data out"=w545:T11)
            n200 = Enqueue Element(queue=w541, element=w538) -> (queue out=w540:refnum<queue>)  [unwired: 2 in, 2 out]
            n201 = Enqueue Element(queue=w547, element=w545) -> (queue out=w544:refnum<queue>, error out=w543:errorcluster)  [unwired: 2 in, 1 out]
          }
          frame Enabled {
          }
        }
      }
    }
    n202 = case shown="True" "Save data" {
      tunnel: w460 -> [w551 w571]
      tunnel: w457 -> [_ w561]
      tunnel: w456 -> [w550 w560]
      frame False {
        n203 = case shown="True" "Purge data" {
          tunnel: w551 -> [_ w554]
          tunnel: w550 -> [_ w553]
          frame False {
          }
          frame True {
            n204 = Flush Queue(queue=w554) -> ()  [unwired: 1 in, 3 out]
            n205 = Flush Queue(queue=w553) -> ()  [unwired: 1 in, 3 out]
          }
        }
      }
      frame True {
        n206 = Flush Queue(queue=w571, error in (no error)=w561) -> (remaining elements=w567:T12)  [unwired: 2 out]
        n207 = Flush Queue(queue=w560, error in (no error)=w561) -> (remaining elements=w559:T3[])  [unwired: 2 out]
        n208 = for {
          tunnel: [w578] -> w570 mode=indexing
          tunnel: [w577] -> w569 mode=indexing
          tunnel: [w576] -> w562 mode=indexing
          tunnel: w567 -> [w575] mode=indexing
          tunnel: w559 -> [w574] mode=indexing
          tunnel: [w573] -> w558 mode=indexing
          tunnel: [w572] -> w557 mode=indexing
          n209 = Unbundle By Name(w575) -> ("Centroid X"=w578:dbl[], "Centroid Y"=w577:dbl[], "Acquired Buffer Number"=w576:u32)
          n210 = Unbundle By Name(w574) -> ("X (IMAQ)"=w573:dbl[], "Y (IMAQ)"=w572:dbl[])
        }
        n211 = Transpose 2D Array(2D array=w570) -> (transposed array=w565:dbl[][])
        n212 = Transpose 2D Array(2D array=w569) -> (transposed array=w564:dbl[][])
        n213 = Transpose 2D Array(2D array=w558) -> (transposed array=w556:dbl[][])
        n214 = Transpose 2D Array(2D array=w557) -> (transposed array=w555:dbl[][])
        n215 = Build Array (concatenate)(w562, w565, w564, w556, w555) -> (w566:dbl[][])
        n216 = Transpose 2D Array(2D array=w566) -> (transposed array=w563:dbl[][])
        n217 = call-poly <vilib>:"Write To Spreadsheet File.vi"("format (%.3f)"="%.9f", "2D data"=w563) -> ()  [unwired: 6 in, 1 out]
      }
    }
    n218 = local read "Stop program"() -> (w478:bool)
  }
  n219 = property on="Show image" class="Bool (strict)"("Visible"=w39) -> ()  [unwired: 2 in, 2 out]
  n220 = property on="ROI size" class="DigNum (strict)"("Visible"=w39) -> ()  [unwired: 2 in, 2 out]
  n221 = property on="Video tracking" class="Bool (strict)"("Visible"=w39) -> ()  [unwired: 2 in, 2 out]
  n222 = property on="Save data" class="Bool"("Visible"=w39) -> ()  [unwired: 2 in, 2 out]
  n223 = property on="Follow traps" class="Bool (strict)"("Visible"=w39) -> ()  [unwired: 2 in, 2 out]
  n224 = property on="Purge data" class="Bool"("Visible"=w39) -> ()  [unwired: 2 in, 2 out]
  n225 = call "FreeGPUandSLM.vi"("error in"=w30) -> ("error out"=w29:errorcluster)  [unwired: 1 out]
  "CUDA/SLM error" <- w29
  n226 = call-poly <vilib>:"Close Input Device.vi"("error in (no error)"=w25, "device ID"=w27) -> ()  [unwired: 9 out]
  n227 = case shown="True" w13 {
    tunnel: w51 -> [_ w585]
    tunnel: w50 -> [w580 w584]
    tunnel: w40 -> [_ w583]
    tunnel: w15 -> [_ w582]
    tunnel: [w580 w581] -> w32
    frame False {
    }
    frame True {
      n228 = case shown="False" w582 {
        tunnel: w585 -> [_ w591]
        tunnel: w584 -> [w588 w590]
        tunnel: [w587 w589] -> w581
        tunnel: w583 -> [w586 _]
        frame False {
          n229 = call <vilib>:"IMAQdx Close Camera.vi"("error in"=w588, "Session In"=w586) -> ("error out"=w587:errorcluster)  [unwired: 9 in]
        }
        frame True {
          n230 = call <vilib>:"IMAQ Close.vi"("error in (no error)"=w590, "IMAQ Session In"=w591) -> ("error out"=w589:errorcluster)  [unwired: 9 in]
        }
      }
    }
  }
  n231 = Merge Errors(w32, w31) -> (w28:errorcluster)
  "NI Vision error" <- w28
  n232 = call "IMAQ Dispose"("Image"=w41) -> ()  [unwired: 5 in, 1 out]
  n233 = for {
    tunnel: w42 -> [w592] mode=indexing
    n234 = call "IMAQ Dispose"("Image"=w592) -> ()  [unwired: 5 in, 1 out]
  }
  n235 = Unbundle By Name(w33) -> ("Contours"=w38:T13)
  n236 = Index Array(array=w38) -> (element=w37:T14)  [unwired: 1 in]
  n237 = flat-sequence {
    tunnel: w29 -> [_]
    tunnel: w28 -> [_]
    frame #0 {
      n238 = local write "Stop program"(FALSE ("Stop program")) -> ()
    }
  }
  n239 = Unbundle By Name(w37) -> ("ROI Type"=w36:u32)
  n240 = Equal?(x=w36, y=u32 1) -> (x = y?=w34:bool)
  n241 = case shown="True" w34 {
    tunnel: w33 -> [_ w594]
    frame False {
    }
    frame True {
      n242 = local write "ROI"(w594) -> ()
    }
  }
